vi "Summer.vi"() -> ()   [LabVIEW 2010]
uses:
  <vilib>/Platform/TimedLoop/XDataNode/XDataNode.xnode
  <vilib>/Platform/TimedLoop/XDataNode/timing_clust.ctl
  <vilib>/Platform/TimedLoop/XDataNode/nitl_modes.ctl
  <vilib>/Platform/TimedLoop/XDataNode/wakeup.ctl
  <vilib>/Platform/TimedLoop/XDataNode/XDNodeRunTimeDep.lvlib
panel:
  out "Waveform Graph":dynamicdata(graph)
  out "data":dbl
  out "Waveform Graph 2":dynamicdata(graph)
  in  "stop":bool
  in  "4Phase (Degrees)":dbl
  in  "4DC Offset":dbl
  in  "4 Amplitude":dbl
  in  "4Frequency (Hz)":dbl
  in  "3 Phase (Degrees)":dbl
  in  "3DC Offset":dbl
  in  "3 Amplitude":dbl
  in  "3Frequency (Hz)":dbl
  in  "2 Phase (Degrees)":dbl
  in  "2 DC Offset":dbl
  in  "2 Amplitude":dbl
  in  "2 Frequency (Hz)":dbl
  in  "1 Phase (Degrees)":dbl
  in  "1 DC Offset":dbl
  in  "1Amplitude":dbl
  in  "1 Frequency (Hz)":dbl
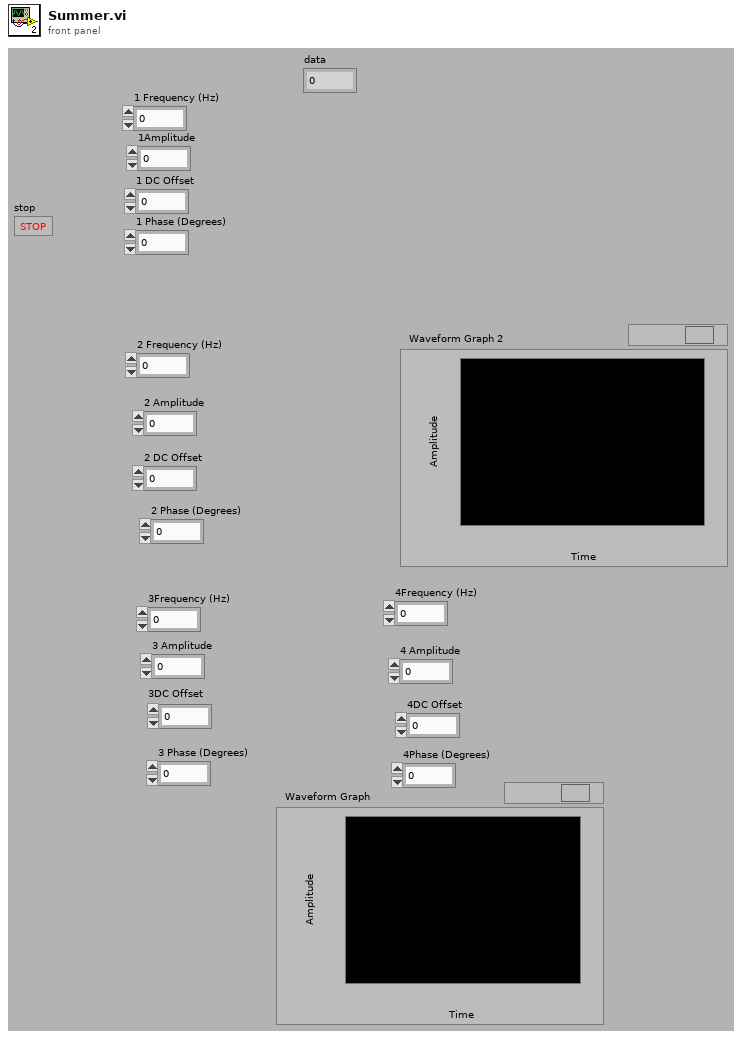
[diagram p1: front panel]
types:
  T1 = typedef "XDNodeRunTimeDep.lvlib/timing_clust.ctl" = cluster{"Expected End [f-1]":u64, "Actual End [f-1]":u64, "Finished Late? [f-1]":bool, "Expected End [i-1]":u64, "Actual End [i-1]":u64, "Finished Late? [i-1]":bool, "Expected Start [i]":u64, "Actual Start [i]":u64, "Expected Start [f]":u64, "Actual Start [f]":u64, "Source Name":string, "Structure Name":string, "Period":i64, "Deadline":i64, "Offset":i64, "Start":i64, "Priority":i32, "Timeout":i32, "Mode":T2, "Wakeup Reason":T3, "Error":errorcluster, "Source Type":string, "Secondary Source Type":string, "Global End Time":u64, "Global Start Time":u64, "Frame Duration":u64, "Iteration Duration":u64, "Assigned CPU":i32, "I/O Scan Engine Mode":u32}
  T2 = typedef "XDNodeRunTimeDep.lvlib/nitl_modes.ctl" = enum32{"No Change", "Process missed periods, maintain original phase", "Discard missed periods, maintain original phase", "Process missed periods, ignore original phase", "Discard missed periods, ignore original phase"}
  T3 = typedef "XDNodeRunTimeDep.lvlib/wakeup.ctl" = enum32{"Normal", "Aborted", "Asynchronous wakeup", "Timing source error", "Timed loop error", "Timeout"}
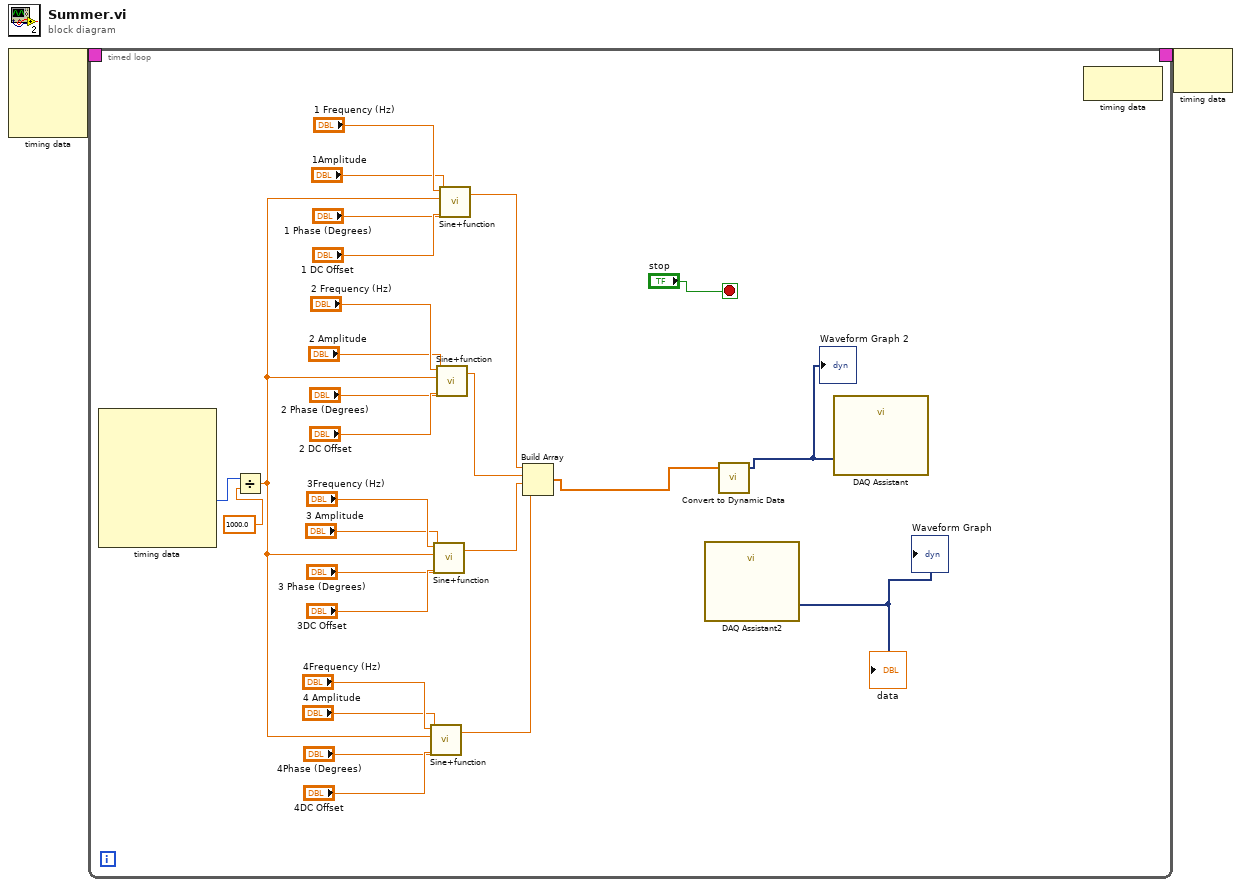
[diagram p0: block diagram]
diagram:
  n1 = node-c288() -> (w2:T1)  [unwired: 4 in]
  n2 = timed-loop {
    timing: w2 -> [_]
    timing-out: [_] -> w1
    stop <- "stop" stop-if-true
    n3 = node-c288() -> (w12:i64)  [unwired: 1 in, 7 out]
    n4 = Divide(x=w12, y=1000.0) -> (x/y=w11:dbl)
    n5 = call "Sine+function.vi"("Frequency (Hz)"="4Frequency (Hz)", "Time (Sec)"=w11, "Amplitude"="4 Amplitude", "DC Offset"="4DC Offset", "Phase (Degrees)"="4Phase (Degrees)") -> ("A*sin(2*pi*f*t+phi)+B"=w8:dbl)  [unwired: 1 in]
    n6 = call "Sine+function.vi"("Frequency (Hz)"="3Frequency (Hz)", "Time (Sec)"=w11, "Amplitude"="3 Amplitude", "DC Offset"="3DC Offset", "Phase (Degrees)"="3 Phase (Degrees)") -> ("A*sin(2*pi*f*t+phi)+B"=w9:dbl)  [unwired: 1 in]
    n7 = call "Sine+function.vi"("Frequency (Hz)"="2 Frequency (Hz)", "Time (Sec)"=w11, "Amplitude"="2 Amplitude", "DC Offset"="2 DC Offset", "Phase (Degrees)"="2 Phase (Degrees)") -> ("A*sin(2*pi*f*t+phi)+B"=w10:dbl)  [unwired: 1 in]
    n8 = call "Sine+function.vi"("Frequency (Hz)"="1 Frequency (Hz)", "Time (Sec)"=w11, "Amplitude"="1Amplitude", "DC Offset"="1 DC Offset", "Phase (Degrees)"="1 Phase (Degrees)") -> ("A*sin(2*pi*f*t+phi)+B"=w5:dbl)  [unwired: 1 in]
    n9 = Build Array(w5, w10, w9, w8) -> (w7:dbl[])
    n10 = call "DAQ Assistant2"() -> ("data"=→"data" →"Waveform Graph":dynamicdata)  [unwired: 17 in, 2 out]
    n11 = call "Convert to Dynamic Data"("Array"=w7) -> ("Dynamic Data Type"=w4:dynamicdata)  [unwired: 3 in]
    "Waveform Graph 2" <- w4
    n12 = call "DAQ Assistant"("data"=w4) -> ()  [unwired: 17 in, 2 out]
    n13 = node-c288() -> ()  [unwired: 1 in, 1 out]
  }
  n14 = node-c288(w1) -> ()  [unwired: 1 out]
